vi "Get XRT-U Angle.vi"(8 "error in (no error)":errorcluster, 11 "Inst.Xeryon-Rotator in":refnum<class "Inst.Xeryon-Rotator.lvclass">) -> (0 "error out":errorcluster, 1 "delimited string":string, 2 "EPOS In Current Units":dbl, 3 "Inst.Xeryon-Rotator out":refnum<class "Inst.Xeryon-Rotator.lvclass">)   [LabVIEW 2019, in "Inst.Xeryon-Rotator.lvclass"]
uses:
  Inst.Xeryon-Rotator.lvclass
  drivers/Class/Controller/Controller.lvclass
  <vilib>/Utility/Data Type/NI_Data Type.lvlib
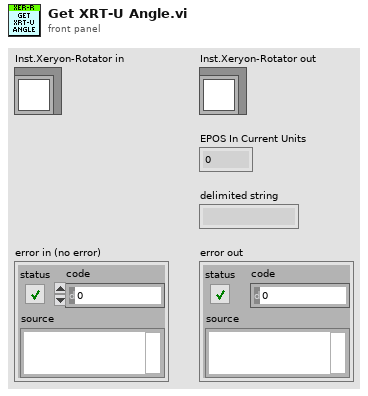
[diagram p1: front panel]
types:
  T1 = cluster{"Index Found":bool, "Left Limit":bool, "Right Limit":bool, "Position Reached":bool}
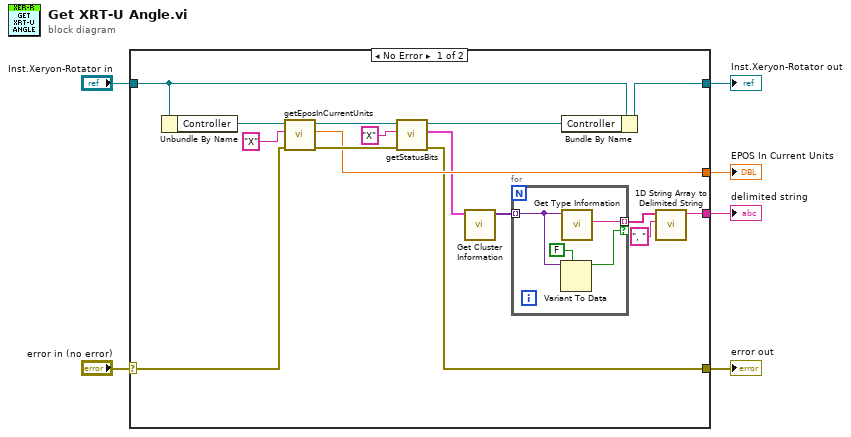
[diagram p0: block diagram]
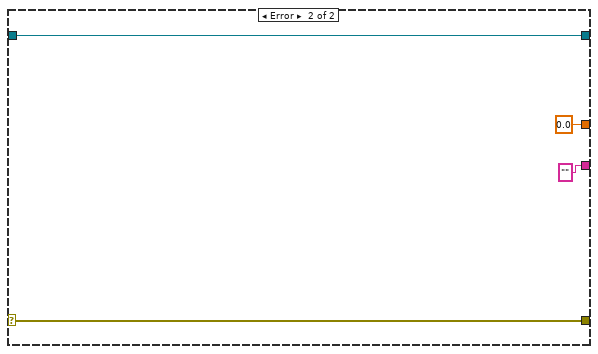
[diagram p2: hidden frame]
diagram:
  n1 = case shown="No Error" "error in (no error)" {
    selector: "error in (no error)" -> [w15 w29]
    tunnel: "Inst.Xeryon-Rotator in" -> [w22 w30]
    tunnel: [w21 w30] -> w2
    tunnel: [w14 0.0 ("EPOS In Current Units")] -> w4
    tunnel: [w10 w29] -> w5
    tunnel: [w8 "" ("delimited string")] -> w6
    frame No Error {
      n2 = Unbundle By Name(w22) -> ("Controller"=w13:refnum<class "Controller.lvclass">)
      n3 = call-dynamic "getEposInCurrentUnits.vi"("error in (no error)"=w15, "Axis Letter"="X", "Controller in"=w13) -> ("error out"=w16:errorcluster, "EPOS In Current Units"=w14:dbl, "Controller out"=w20:refnum<class "Controller.lvclass">)  [unwired: 6 in]
      n4 = call-dynamic "getStatusBits.vi"("error in (no error)"=w16, "Axis Letter"="X", "Controller in"=w20) -> ("error out"=w10:errorcluster, "StatusBits"=w12:T1, "Controller out"=w19:refnum<class "Controller.lvclass">)  [unwired: 6 in]
      n5 = call <vilib>:"Get Cluster Information.vi"("variant"=w12) -> ("cluster elements"=w11:variant[])  [unwired: 9 in, 1 out]
      n6 = for {
        tunnel: w11 -> [w26] mode=indexing
        tunnel: [w24] -> w7 mode=indexing if=w23
        n7 = Variant To Data(type=FALSE, Variant=w26) -> (data=w23:bool)  [unwired: 1 in, 1 out]
        n8 = call <vilib>:"Get Type Information.vi"("variant"=w26) -> ("name"=w24:string)  [unwired: 6 in, 4 out]
      }
      n9 = Bundle By Name(cluster=w22, "Controller"=w19) -> (w21:refnum<class "Inst.Xeryon-Rotator.lvclass">)
      n10 = call <vilib>:"1D String Array to Delimited String.vi"("delimiter"=", ", "string array"=w7) -> ("delimited string"=w8:string)  [unwired: 9 in]
    }
    frame Error {
    }
  }
  "delimited string" <- w6
  "error out" <- w5
  "EPOS In Current Units" <- w4
  "Inst.Xeryon-Rotator out" <- w2
